vi "PRAT Extract Data Convert to 1DBL.vi"(8 "Error In":errorcluster, 10 "Extract Column":i32, 11 "Full Cycle Data":string[][](array[string])) -> (0 "Error Out":errorcluster, 3 "DBL":dbl[](array[numeric]))   [LabVIEW 2016]
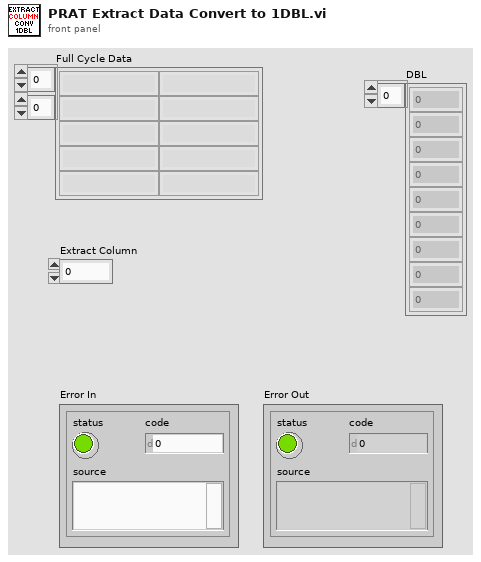
[diagram p1: front panel]
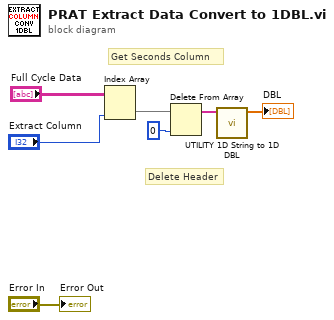
[diagram p0: block diagram]
diagram:
  # "Delete Header"
  # "Get Seconds Column"
  n1 = Index Array(array="Full Cycle Data", index (col)="Extract Column") -> (element=w5:string[])  [unwired: 1 in]
  n2 = Delete From Array(array=w5, index=0) -> (array with subset deleted=w3:string[])  [unwired: 1 in, 1 out]
  n3 = call "UTILITY 1D String to 1D DBL.vi"("Save Data"=w3) -> ("DBL"=→"DBL":dbl[])  [unwired: 10 in]
  "Error Out" <- "Error In"
